vi "Get Directories with Pattern.vi"(8 "error in (no error)":errorcluster caption="错误输入（无错误）", 9 "searchPattern":string, 10 "Directory":path) -> (0 "error out":errorcluster caption="错误输出", 2 "Directories":path[](array[path]))   [LabVIEW 2012, in "Directory.lvclass"]
uses:
  Directory.lvclass
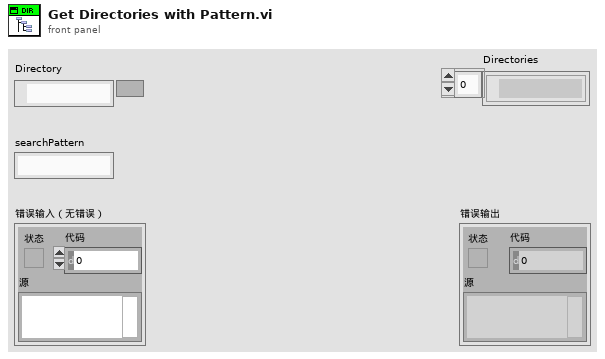
[diagram p1: front panel]
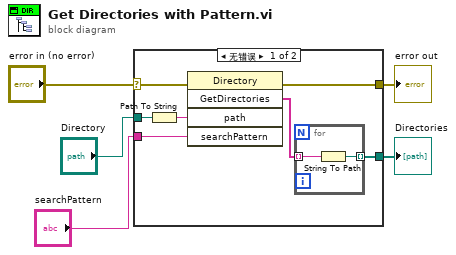
[diagram p0: block diagram]
diagram:
  n1 = case shown="无错误" "error in (no error)" {
    selector: "error in (no error)" -> [w12 w15]
    tunnel: [w11 w15] -> w4
    tunnel: "Directory" -> [w10 _]
    tunnel: [w7 _] -> w2
    tunnel: "searchPattern" -> [w6 _]
    frame No Error {
      n2 = Path To String(path=w10) -> (string=w9:string)
      n3 = invoke on="调用节点" class="Directory" method="GetDirectories"(error in=w12, "path"=w9, "searchPattern"=w6) -> (error out=w11:errorcluster, "GetDirectories"=w8:string[])  [unwired: 2 in, 3 out]
      n4 = for {
        tunnel: w8 -> [w14] mode=indexing
        tunnel: [w13] -> w7 mode=indexing
        n5 = String To Path(string=w14) -> (path=w13:path)
      }
    }
    frame Error {
    }
  }
  "error out" <- w4
  "Directories" <- w2
